vi "MapPixelSpace.vi"(1 "angle (deg)":dbl) -> (0 "spacemapout":dbl)   [LabVIEW 2010]
panel:
  # "Pixel space undistortion algorithm.\nThis subVI is used with simulation sonar to  turn pixel distances into undistorted linear distance.\nDo so by curve fitting angle versus distance for one block traveled\nfor each 0ctant of 45 degrees.\nDoing so, unwarps pixel space into linear x,y space."
  # "1 block move at 45 equals 1.414"
  # "1 move in x or y equals 1"
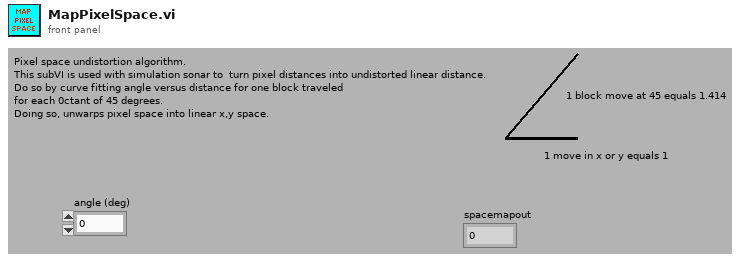
[diagram p1: front panel]
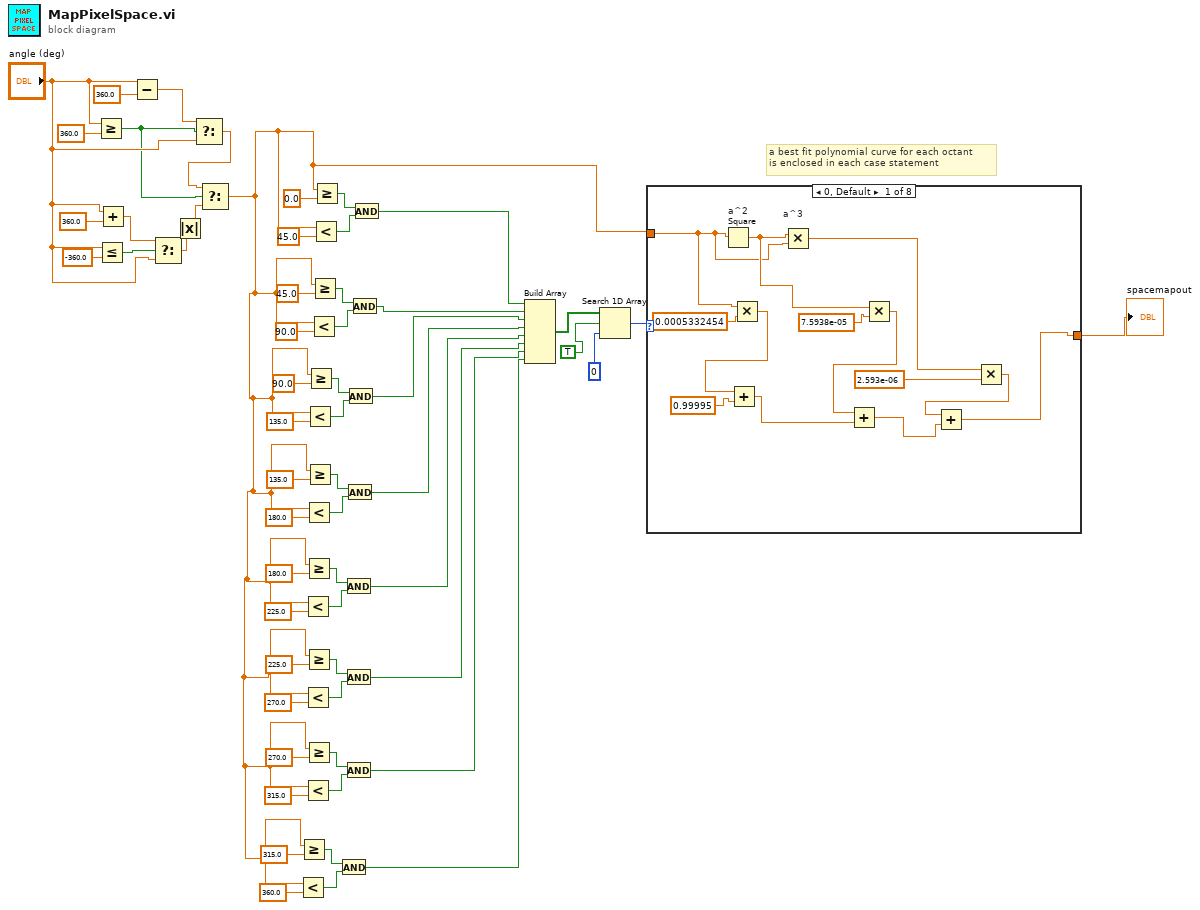
[diagram p0: block diagram]
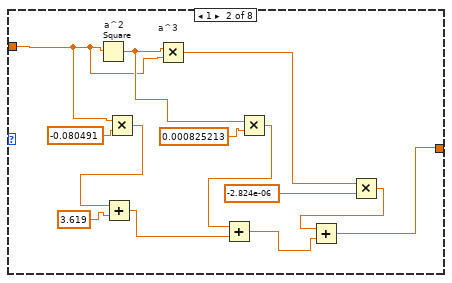
[diagram p2: hidden frame]
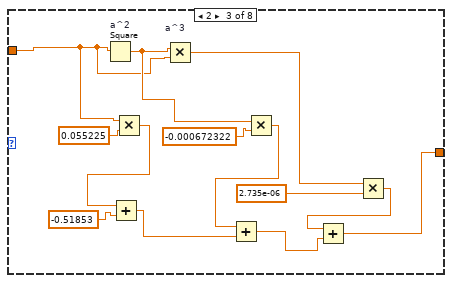
[diagram p3: hidden frame]
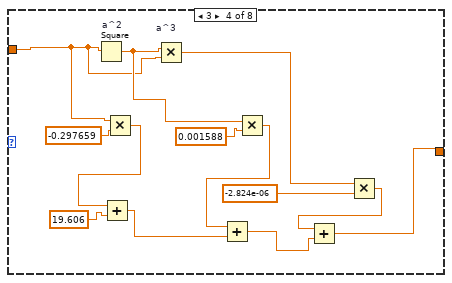
[diagram p4: hidden frame]
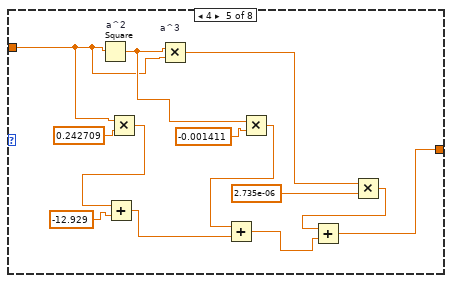
[diagram p5: hidden frame]
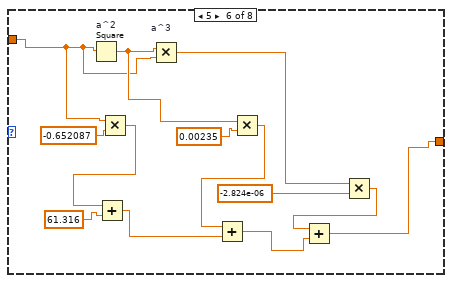
[diagram p6: hidden frame]
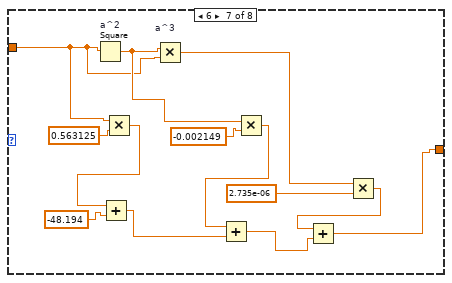
[diagram p7: hidden frame]
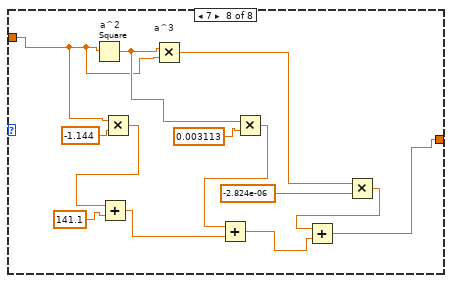
[diagram p8: hidden frame]
diagram:
  # "a best fit polynomial curve for each octant \nis enclosed in each case statement"
  n1 = Greater Or Equal?(x="angle (deg)", y=360.0) -> (x >= y?=w2:bool)
  n2 = Less Or Equal?(x="angle (deg)", y=-360.0) -> (x <= y?=w7:bool)
  n3 = Add(x="angle (deg)", y=360.0) -> (x+y=w8:dbl)
  n4 = Subtract(x="angle (deg)", y=360.0) -> (x-y=w11:dbl)
  n5 = Select(t=w8, s=w7, f="angle (deg)") -> (s? t:f=w3:dbl)
  n6 = Absolute Value(x=w3) -> (abs(x)=w1:dbl)
  n7 = Select(t=w11, s=w2, f="angle (deg)") -> (s? t:f=w4:dbl)
  n8 = Select(t=w4, s=w2, f=w1) -> (s? t:f=w5:dbl)
  n9 = Less?(x=w5, y=360.0) -> (x < y?=w23:bool)
  n10 = Greater Or Equal?(x=w5, y=315.0) -> (x >= y?=w22:bool)
  n11 = Less?(x=w5, y=225.0) -> (x < y?=w36:bool)
  n12 = Less?(x=w5, y=270.0) -> (x < y?=w31:bool)
  n13 = Less?(x=w5, y=315.0) -> (x < y?=w28:bool)
  n14 = Less?(x=w5, y=180.0) -> (x < y?=w39:bool)
  n15 = Greater Or Equal?(x=w5, y=180.0) -> (x >= y?=w37:bool)
  n16 = Greater Or Equal?(x=w5, y=225.0) -> (x >= y?=w30:bool)
  n17 = Greater Or Equal?(x=w5, y=270.0) -> (x >= y?=w29:bool)
  n18 = Less?(x=w5, y=135.0) -> (x < y?=w44:bool)
  n19 = Greater Or Equal?(x=w5, y=135.0) -> (x >= y?=w38:bool)
  n20 = Greater Or Equal?(x=w5, y=90.0) -> (x >= y?=w45:bool)
  n21 = Less?(x=w5, y=90.0) -> (x < y?=w47:bool)
  n22 = Greater Or Equal?(x=w5, y=45.0) -> (x >= y?=w46:bool)
  n23 = Less?(x=w5, y=45.0) -> (x < y?=w55:bool)
  n24 = Greater Or Equal?(x=w5, y=0.0) -> (x >= y?=w56:bool)
  n25 = And(x=w22, y=w23) -> (x .and. y?=w15:bool)
  n26 = And(x=w37, y=w36) -> (x .and. y?=w18:bool)
  n27 = And(x=w30, y=w31) -> (x .and. y?=w17:bool)
  n28 = And(x=w29, y=w28) -> (x .and. y?=w16:bool)
  n29 = And(x=w38, y=w39) -> (x .and. y?=w19:bool)
  n30 = And(x=w45, y=w44) -> (x .and. y?=w20:bool)
  n31 = And(x=w46, y=w47) -> (x .and. y?=w21:bool)
  n32 = And(x=w56, y=w55) -> (x .and. y?=w52:bool)
  n33 = Build Array "Build Array"(w52, w21, w20, w19, w18, w17, w16, w15) -> (w51:bool[])
  n34 = Search 1D Array(1D array=w51, element=TRUE, start index (0)=0) -> (index of element=w58:i32)
  n35 = case shown="0, Default" w58 {
    tunnel: w5 -> [w67 w73 w86 w99 w112 w125 w138 w151]
    tunnel: [w59 w72 w85 w98 w111 w124 w137 w150] -> w14
    frame 0, Default {
      n36 = Square "a^2"(x=w67) -> (x^2=w71:dbl)
      n37 = Multiply(x=w67, y=0.0005332454) -> (x*y=w66:dbl)
      n38 = Add(x=w66, y=0.99995) -> (x+y=w64:dbl)
      n39 = Multiply "a^3"(x=w71, y=w67) -> (x*y=w70:dbl)
      n40 = Multiply(x=w71, y=7.5938e-05) -> (x*y=w63:dbl)
      n41 = Add(x=w63, y=w64) -> (x+y=w61:dbl)
      n42 = Multiply(x=w70, y=2.593e-06) -> (x*y=w60:dbl)
      n43 = Add(x=w60, y=w61) -> (x+y=w59:dbl)
    }
    frame 1 {
      n44 = Square "a^2"(x=w73) -> (x^2=w84:dbl)
      n45 = Multiply(x=w73, y=-0.080491) -> (x*y=w80:dbl)
      n46 = Add(x=w80, y=3.619) -> (x+y=w78:dbl)
      n47 = Multiply "a^3"(x=w84, y=w73) -> (x*y=w83:dbl)
      n48 = Multiply(x=w84, y=0.000825213) -> (x*y=w77:dbl)
      n49 = Add(x=w77, y=w78) -> (x+y=w75:dbl)
      n50 = Multiply(x=w83, y=-2.824e-06) -> (x*y=w74:dbl)
      n51 = Add(x=w74, y=w75) -> (x+y=w72:dbl)
    }
    frame 2 {
      n52 = Square "a^2"(x=w86) -> (x^2=w97:dbl)
      n53 = Multiply(x=w86, y=0.055225) -> (x*y=w93:dbl)
      n54 = Add(x=w93, y=-0.51853) -> (x+y=w91:dbl)
      n55 = Multiply "a^3"(x=w97, y=w86) -> (x*y=w96:dbl)
      n56 = Multiply(x=w97, y=-0.000672322) -> (x*y=w90:dbl)
      n57 = Add(x=w90, y=w91) -> (x+y=w88:dbl)
      n58 = Multiply(x=w96, y=2.735e-06) -> (x*y=w87:dbl)
      n59 = Add(x=w87, y=w88) -> (x+y=w85:dbl)
    }
    frame 3 {
      n60 = Square "a^2"(x=w99) -> (x^2=w110:dbl)
      n61 = Multiply(x=w99, y=-0.297659) -> (x*y=w106:dbl)
      n62 = Add(x=w106, y=19.606) -> (x+y=w104:dbl)
      n63 = Multiply "a^3"(x=w110, y=w99) -> (x*y=w109:dbl)
      n64 = Multiply(x=w110, y=0.001588) -> (x*y=w103:dbl)
      n65 = Add(x=w103, y=w104) -> (x+y=w101:dbl)
      n66 = Multiply(x=w109, y=-2.824e-06) -> (x*y=w100:dbl)
      n67 = Add(x=w100, y=w101) -> (x+y=w98:dbl)
    }
    frame 4 {
      n68 = Square "a^2"(x=w112) -> (x^2=w123:dbl)
      n69 = Multiply(x=w112, y=0.242709) -> (x*y=w119:dbl)
      n70 = Add(x=w119, y=-12.929) -> (x+y=w117:dbl)
      n71 = Multiply "a^3"(x=w123, y=w112) -> (x*y=w122:dbl)
      n72 = Multiply(x=w123, y=-0.001411) -> (x*y=w116:dbl)
      n73 = Add(x=w116, y=w117) -> (x+y=w114:dbl)
      n74 = Multiply(x=w122, y=2.735e-06) -> (x*y=w113:dbl)
      n75 = Add(x=w113, y=w114) -> (x+y=w111:dbl)
    }
    frame 5 {
      n76 = Square "a^2"(x=w125) -> (x^2=w136:dbl)
      n77 = Multiply(x=w125, y=-0.652087) -> (x*y=w132:dbl)
      n78 = Add(x=w132, y=61.316) -> (x+y=w130:dbl)
      n79 = Multiply "a^3"(x=w136, y=w125) -> (x*y=w135:dbl)
      n80 = Multiply(x=w136, y=0.00235) -> (x*y=w129:dbl)
      n81 = Add(x=w129, y=w130) -> (x+y=w127:dbl)
      n82 = Multiply(x=w135, y=-2.824e-06) -> (x*y=w126:dbl)
      n83 = Add(x=w126, y=w127) -> (x+y=w124:dbl)
    }
    frame 6 {
      n84 = Square "a^2"(x=w138) -> (x^2=w149:dbl)
      n85 = Multiply(x=w138, y=0.563125) -> (x*y=w145:dbl)
      n86 = Add(x=w145, y=-48.194) -> (x+y=w143:dbl)
      n87 = Multiply "a^3"(x=w149, y=w138) -> (x*y=w148:dbl)
      n88 = Multiply(x=w149, y=-0.002149) -> (x*y=w142:dbl)
      n89 = Add(x=w142, y=w143) -> (x+y=w140:dbl)
      n90 = Multiply(x=w148, y=2.735e-06) -> (x*y=w139:dbl)
      n91 = Add(x=w139, y=w140) -> (x+y=w137:dbl)
    }
    frame 7 {
      n92 = Square "a^2"(x=w151) -> (x^2=w162:dbl)
      n93 = Multiply(x=w151, y=-1.144) -> (x*y=w158:dbl)
      n94 = Add(x=w158, y=141.1) -> (x+y=w156:dbl)
      n95 = Multiply "a^3"(x=w162, y=w151) -> (x*y=w161:dbl)
      n96 = Multiply(x=w162, y=0.003113) -> (x*y=w155:dbl)
      n97 = Add(x=w155, y=w156) -> (x+y=w153:dbl)
      n98 = Multiply(x=w161, y=-2.824e-06) -> (x*y=w152:dbl)
      n99 = Add(x=w152, y=w153) -> (x+y=w150:dbl)
    }
  }
  "spacemapout" <- w14
